vi "ULS Shift.vi"   [LabVIEW 2016]
uses:
  Class/IFD/IFD.lvclass
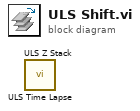
[diagram p0: block diagram]
diagram:
  n1 = call "ULS Time Lapse.vi"() -> ()  [unwired: 10 in, 2 out]
  n2 = call "ULS Z Stack.vi"() -> ()  [unwired: 10 in, 2 out]
